vi "03052013A.vi"() -> ()   [LabVIEW 2012]
panel:
  out "Waveform Chart":cluster{i32, "Elapsed Time (s)":dbl, dbl}(graph)
  in  "access (0:read/write)":enum16{"read/write", "read-only", "write-only"}(ring)
  out "output cluster":cluster{string, string, string}
  in  "operation (0:open) 2":T1(ring)
  in  "file path (use dialog) 2":path
  in  "Knob":dbl(knob)=250.0 scale=0.0..1000.0
  out "Data Panel":T2 {"Elapsed Time (s)" format="%#_5f"}
  out "error out":errorcluster
  out "Array":dbl[][](array[numeric])
  in  "stop":bool
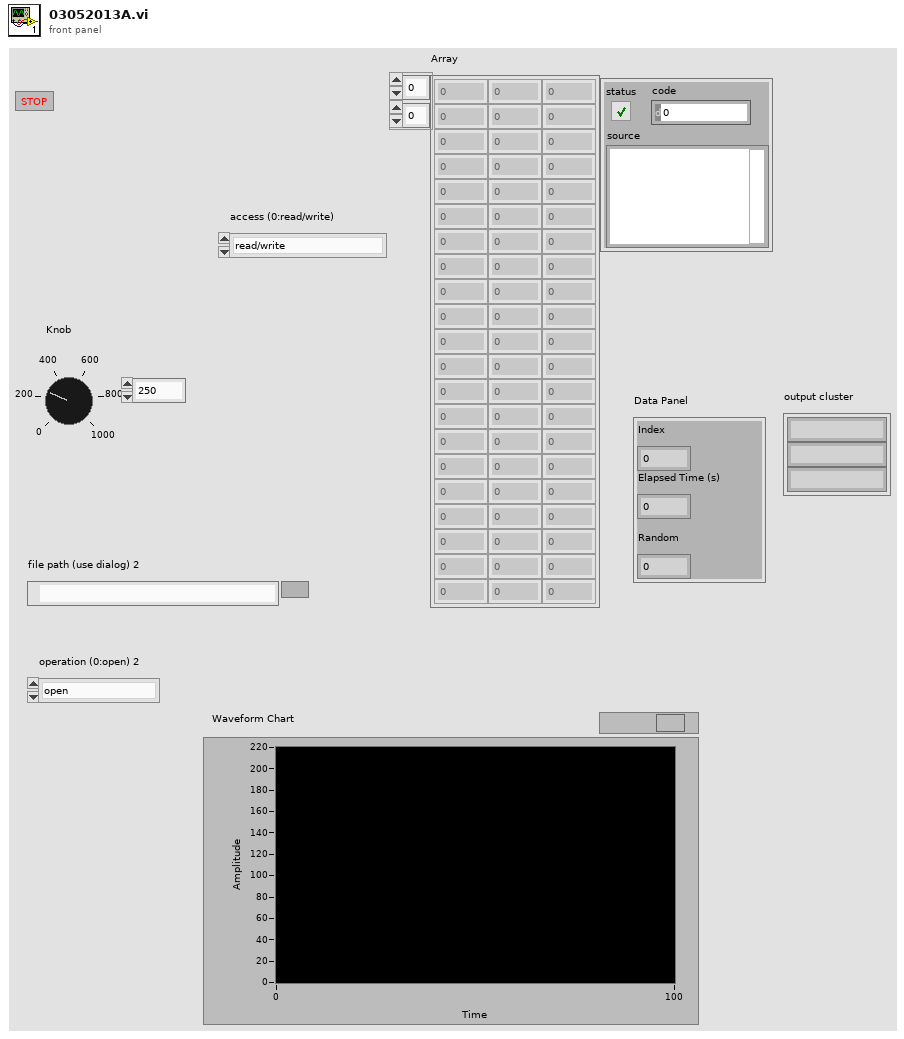
[diagram p1: front panel]
types:
  T1 = enum16{"open", "replace", "create", "open or create", "replace or create", "replace or create with confirmation"}
  T2 = cluster{"Index":i32, "Elapsed Time (s)":dbl, "Random":dbl}
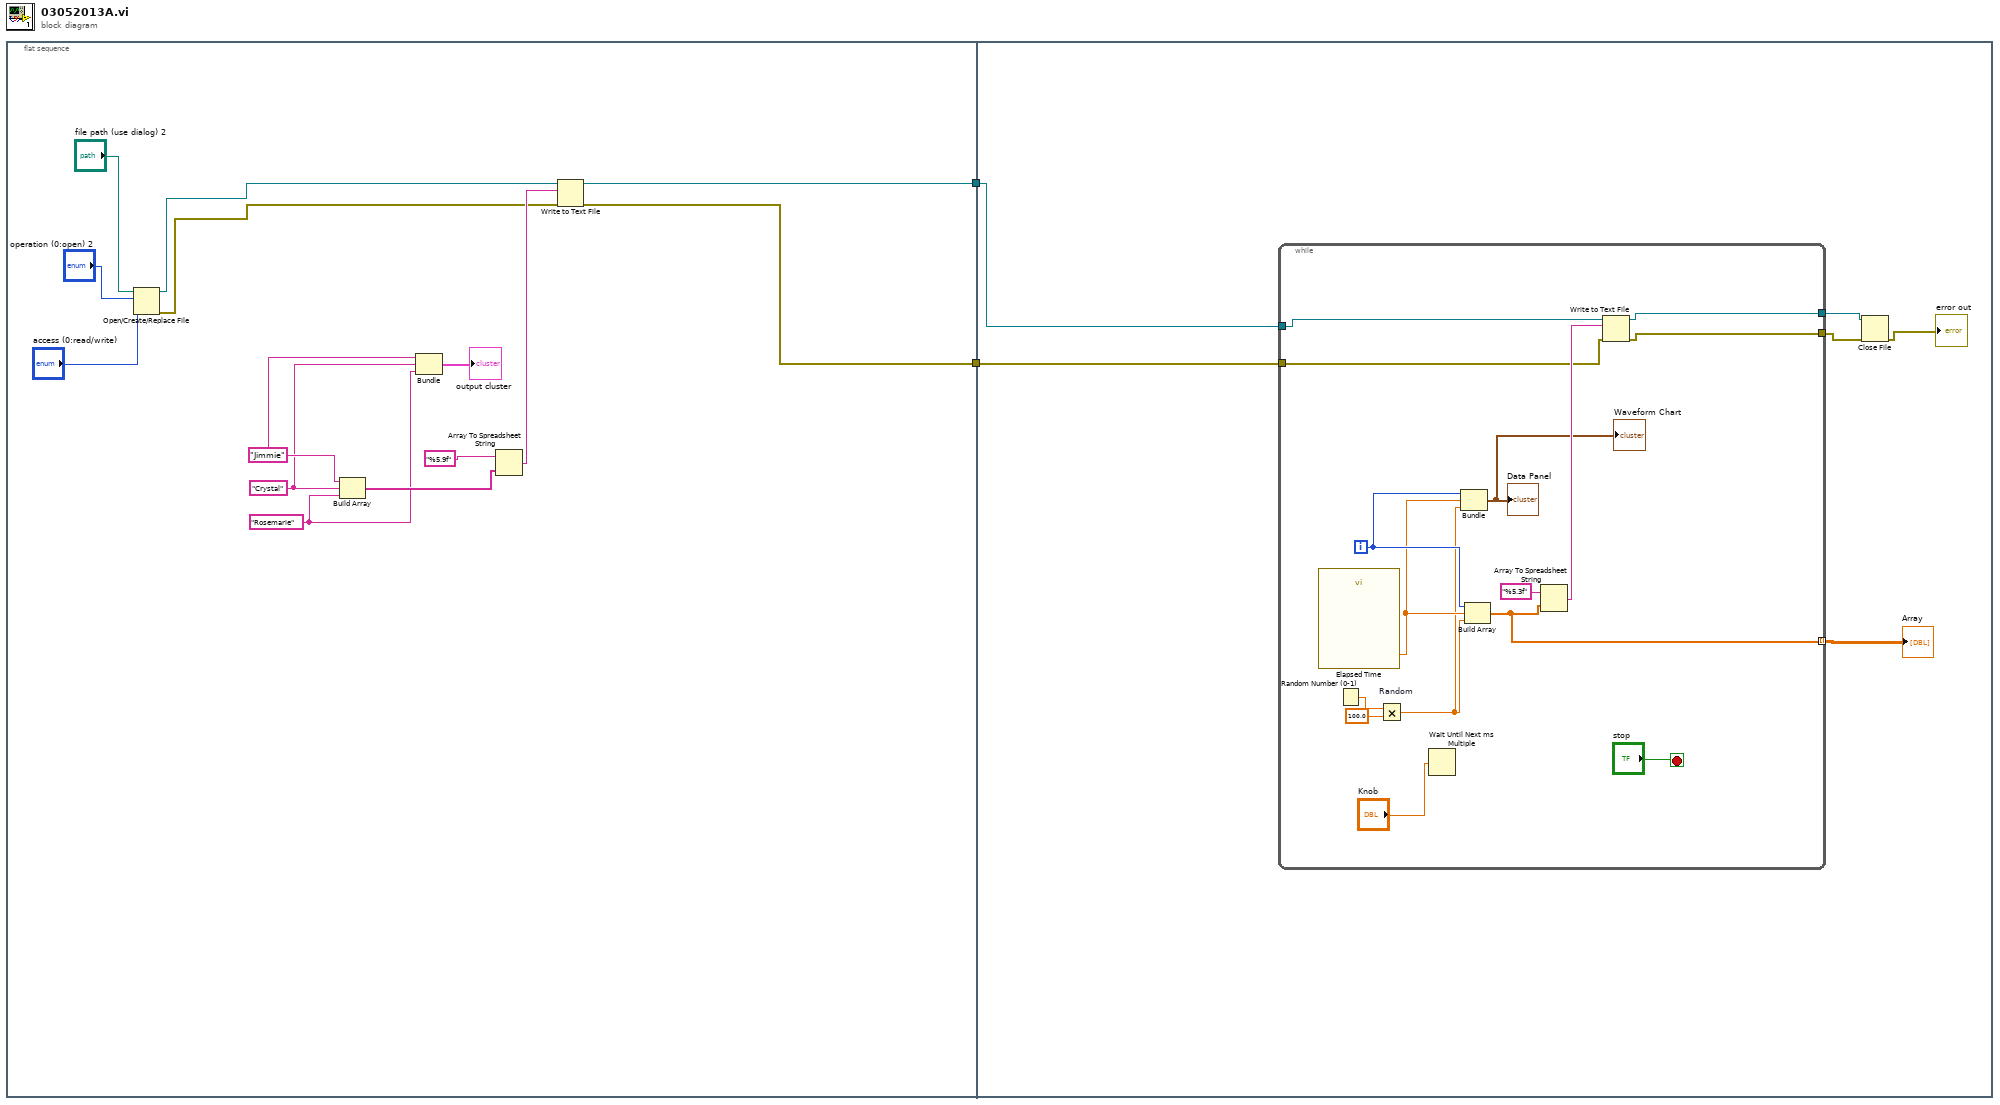
[diagram p0: block diagram]
diagram:
  n1 = flat-sequence {
    tunnel: [w4] -> w2
    tunnel: [w3] -> w1
    tunnel: w2 -> [w18]
    tunnel: w1 -> [w17]
    frame #0 {
      w8 = "Crystal"
      w7 = "Rosemarie"
      w9 = "Jimmie"
      n2 = Open/Create/Replace File(file path (use dialog)="file path (use dialog) 2", operation (0:open)="operation (0:open) 2", access (0:read/write)="access (0:read/write)") -> (refnum out=w12:refnum<file>, error out=w11:errorcluster)  [unwired: 3 in, 1 out]
      n3 = Build Array(w9, w8, w7) -> (w10:string[])
      n4 = Bundle(w9, w8, w7) -> (→"output cluster":cluster{string, string, string})  [unwired: 1 in]
      n5 = Array To Spreadsheet String(array=w10, 3:"%5.9f" ("format string")) -> (spreadsheet string=w16:string)  [unwired: 1 in]
      n6 = Write to Text File(file (use dialog)=w12, text=w16, error in=w11) -> (refnum out=w4:refnum<file>, error out=w3:errorcluster)  [unwired: 1 in, 1 out]
    }
    frame #1 {
      n7 = while {
        tunnel: [w32] -> w20
        tunnel: [w31] -> w21
        tunnel: [w30] -> w22 mode=indexing
        tunnel: w18 -> [w25]
        tunnel: w17 -> [w24]
        i -> [w29]
        stop <- "stop" stop-if-true
        n8 = call "Elapsed Time"() -> ("Elapsed Time (s)"=w28:dbl)  [unwired: 12 in, 7 out]
        n9 = Random Number (0-1)() -> (number: 0 to 1=w36:dbl)
        n10 = Multiply "Random"(x=w36, y=100.0) -> (x*y=w27:dbl)
        n11 = Wait Until Next ms Multiple(millisecond multiple="Knob") -> ()  [unwired: 1 out]
        n12 = Bundle(w29, "Elapsed Time (s)"=w28, w27) -> (→"Data Panel" →"Waveform Chart":cluster{i32, "Elapsed Time (s)":dbl, dbl})  [unwired: 1 in]
        n13 = Build Array(w29, w28, w27) -> (w30:dbl[])
        n14 = Array To Spreadsheet String(array=w30, 3:"%5.3f" ("format string")) -> (spreadsheet string=w33:string)  [unwired: 1 in]
        n15 = Write to Text File(file (use dialog)=w25, text=w33, error in=w24) -> (refnum out=w31:refnum<file>, error out=w32:errorcluster)  [unwired: 1 in, 1 out]
      }
      "Array" <- w22
      n16 = Close File(refnum=w21, error in=w20) -> (error out=→"error out":errorcluster)  [unwired: 1 out]
    }
  }
